vi "Заключение.vi"() -> ()   [LabVIEW 2017]
panel:
  in  "textToSpeak":string="Уважаемые коллеги, благодарим за внимание!\nМы надеемся, что на наших занятиях вы узнали кое-что новое и интересное.\nЖелаем вам всего доброго. \nУвидимся!"
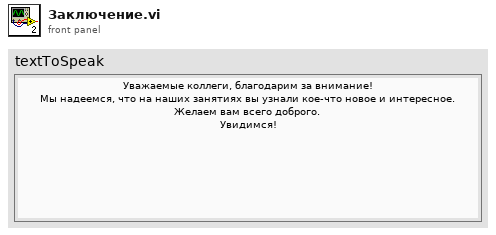
[diagram p1: front panel]
types:
  T1 = typedef "LVDateTimeRec.ctl" = cluster{"fractional second":dbl, "second":i32, "minute":i32, "hour":i32, "day of month":i32, "month":i32, "year":i32, "day of week":i32, "day of year":i32, "DST":i32}
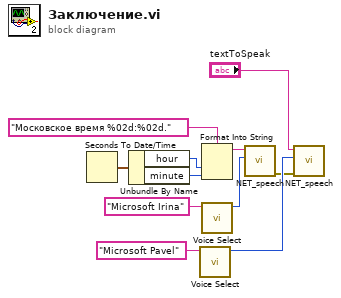
[diagram p0: block diagram]
diagram:
  n1 = Seconds To Date/Time() -> (date time rec=w10:T1)  [unwired: 2 in]
  n2 = Unbundle By Name(w10) -> ("hour"=w8:i32, "minute"=w7:i32)
  n3 = call "Voice Select.vi"("Voice name"="Microsoft Pavel") -> ("Voice"=w4:i32)  [unwired: 10 in]
  n4 = Format Into String(format string="Московское время %02d:%02d.", w8, w7) -> (resulting string=w6:string)  [unwired: 2 in, 1 out]
  n5 = call "Voice Select.vi"("Voice name"="Microsoft Irina") -> ("Voice"=w11:i32)  [unwired: 10 in]
  n6 = call "NET_speech.vi"("Голос"=w11, "textToSpeak"=w6) -> ("error out"=w3:errorcluster)  [unwired: 1 in, 8 out]
  n7 = call "NET_speech.vi"("error in (no error)"=w3, "Голос"=w4, "textToSpeak"="textToSpeak") -> ()  [unwired: 9 out]
